vi "8XY4.vi"(11 "Variables and Memory in":T1 {"GFX" format="%02x"}) -> (3 "Variables and Memory out":T1 {"GFX" format="%02x"})   [LabVIEW 2021]
uses:
  Controls/ClusterF.ctl
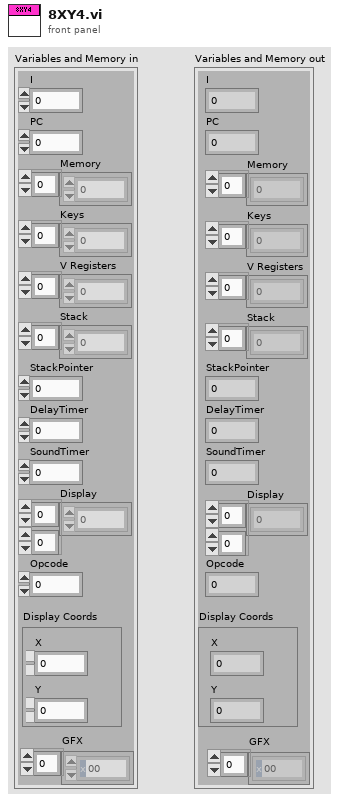
[diagram p1: front panel]
types:
  T1 = typedef "ClusterF.ctl" = cluster{"I":u16, "PC":u16, "Memory":u8[], "Keys":u8[], "V Registers":u8[], "Stack":u16[], "StackPointer":u16, "DelayTimer":u8, "SoundTimer":u8, "Display":u8[][], "Opcode":u16, "Display Coords":cluster{"X":u8, "Y":u8}, "GFX":u8[]}
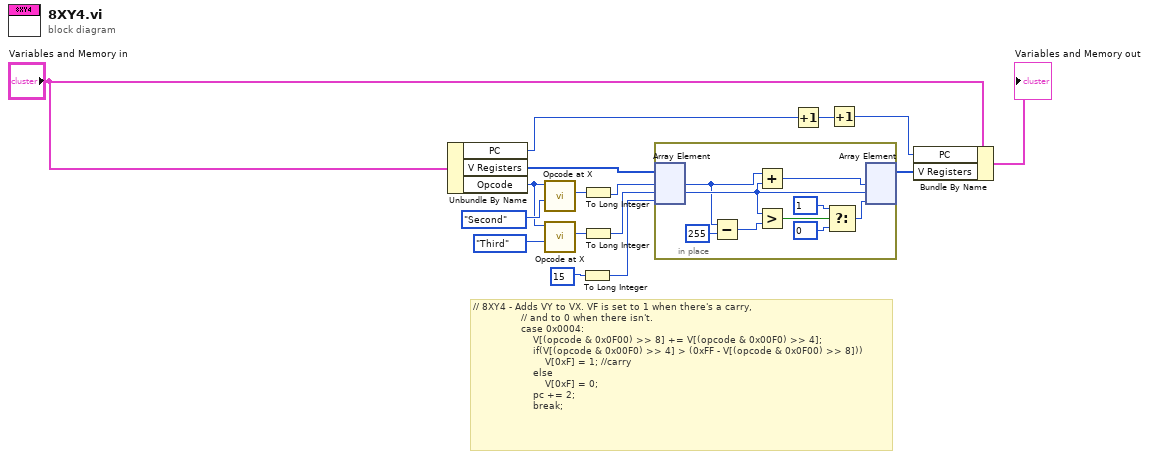
[diagram p0: block diagram]
diagram:
  # "// 8XY4 - Adds VY to VX. VF is set to 1 when there's a carry,\n                // and to 0 when there isn't.\n                case 0x0004:\n                    V[(opcode & 0x0F00) >> 8] += V[(opcode & 0x00F0) >> 4];\n                    if(V[(opcode & 0x00F0) >> 4] > (0xFF - V[(opcode & 0x0F00) >> 8]))\n                        V[0xF] = 1; //carry\n                    else\n                        V[0xF] = 0;\n                    pc += 2;\n                    break;"
  n1 = Unbundle By Name("Variables and Memory in") -> ("PC"=w3:u16, "V Registers"=w13:u8[], "Opcode"=w6:u16)
  n2 = call "Opcode at X.vi"("X Position"=enum16{"First", "Second", "Third", "Fourth"}."Second", "Opcode"=w6) -> ("Opcode at X Position (U8)"=w10:u8)  [unwired: 9 in]
  n3 = call "Opcode at X.vi"("X Position"=enum16{"First", "Second", "Third", "Fourth"}."Third", "Opcode"=w6) -> ("Opcode at X Position (U8)"=w9:u8)  [unwired: 9 in]
  n4 = To Long Integer(number=15) -> (32bit integer=w16:i32)
  n5 = To Long Integer(number=w10) -> (32bit integer=w11:i32)
  n6 = To Long Integer(number=w9) -> (32bit integer=w15:i32)
  n7 = in-place {
    n8 = in-place-array #1(w13, w11, w15, w16) -> (w18:u8, w20:u8)  [unwired: 1 out]
    n9 = Subtract(x=w18, y=u8 255) -> (x-y=w17:u8)
    n10 = Add(x=w18, y=w20) -> (x+y=w25:u8)
    n11 = Greater?(x=w20, y=w17) -> (0:w24:bool)
    n12 = Select(t=u8 1, s=w24, f=u8 0) -> (s? t:f=w21:u8)
    n13 = in-place-array #1(w25, w20, w21) -> (w12:u8[])  [unwired: 3 out]
  }
  n14 = Increment(x=w3) -> (x+1=w4:u16)
  n15 = Increment(x=w4) -> (x+1=w5:u16)
  n16 = Bundle By Name(cluster="Variables and Memory in", "PC"=w5, "V Registers"=w12) -> (→"Variables and Memory out":T1)
